vi "Execute.vi"(8 "error in (no error)":errorcluster, 10 "Notify Plugin Slide Completed in":refnum<class "Notify Plugin Slide Completed.lvclass">, 11 "Plugin Handler Shifter Data Definition":T1) -> (0 "error out":errorcluster, 1 "Stop?":bool, 2 "Plugin Generic Command out":refnum<class "Plugin Handler Command.lvclass">, 3 "Plugin Handler Shifter Data Out":T1)   [LabVIEW 2011, in "Notify Plugin Slide Completed.lvclass"]
uses:
  Notify Plugin Slide Completed.lvclass
  Plugin Handler Command.lvclass
  Plugin Strict Type Definitions/Plugin Handler Shifter Data Definition.ctl
  Parent Plugin Definition/Plugin Template/Generic Plugin.lvclass
  Plugin Strict Type Definitions/Plugin Configuration Information.ctl
  User Interface/UI Command Manager/UI Command Manager.lvclass
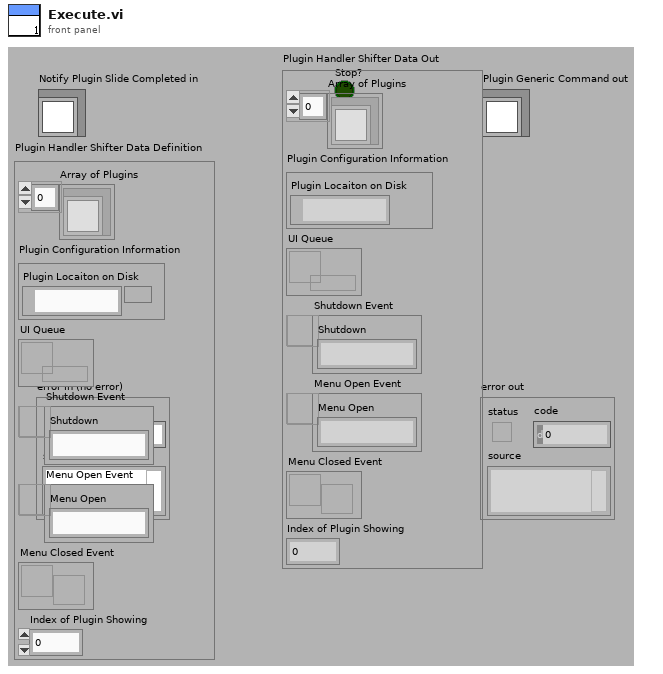
[diagram p1: front panel]
types:
  T1 = typedef "Plugin Handler Shifter Data Definition.ctl" = cluster{"Array of Plugins":refnum<class "Generic Plugin.lvclass">[], "Plugin Configuration Information":T2, "UI Queue":refnum<queue>, "Shutdown Event":refnum<user-event>, "Menu Open Event":refnum<user-event>, "Menu Closed Event":refnum<user-event>, "Index of Plugin Showing":i32}
  T2 = typedef "Plugin Configuration Information.ctl" = cluster{"Plugin Locaiton on Disk":path}
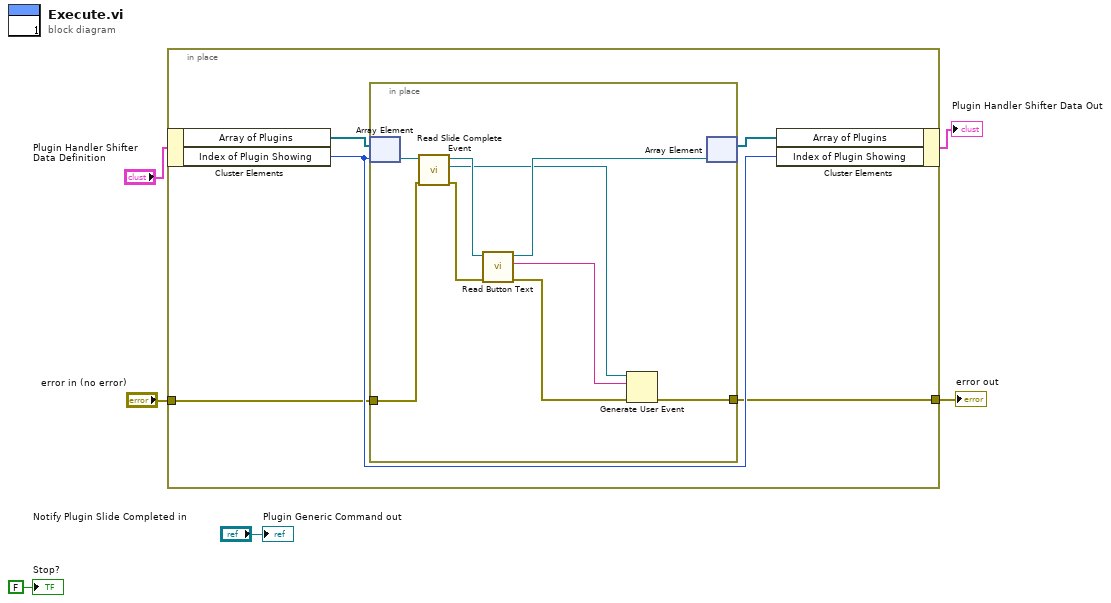
[diagram p0: block diagram]
diagram:
  n1 = in-place {
    in-place-border: "error in (no error)" -> [w8]
    in-place-border: [w7] -> w3
    n2 = in-place-cluster #1("Plugin Handler Shifter Data Definition") -> ("Array of Plugins"=w11:refnum<class "Generic Plugin.lvclass">[], "Index of Plugin Showing"=w9:i32)
    n3 = in-place {
      in-place-border: w8 -> [w17]
      in-place-border: [w12] -> w7
      n4 = in-place-array #2(w11, w9) -> (w20:refnum<class "Generic Plugin.lvclass">)
      n5 = call "Read Slide Complete Event.vi"("error in (no error)"=w17, "Generic Plugin in"=w20) -> ("error out"=w16:errorcluster, "Slide Complete Event"=w14:refnum<user-event>, "Generic Plugin out"=w19:refnum<class "Generic Plugin.lvclass">)  [unwired: 7 in]
      n6 = call-dynamic "Read Button Text.vi"("error in (no error)"=w16, "Generic Plugin in"=w19) -> ("error out"=w13:errorcluster, "Button Text"=w15:string, "Generic Plugin out"=w18:refnum<class "Generic Plugin.lvclass">)  [unwired: 7 in]
      n7 = Generate User Event(user event=w14, event data cluster=w15, error in=w13) -> (error out=w12:errorcluster)  [unwired: 1 out]
      n8 = in-place-array #2(w18) -> (w10:refnum<class "Generic Plugin.lvclass">[])  [unwired: 1 out]
    }
    n9 = in-place-cluster #1("Array of Plugins"=w10, "Index of Plugin Showing"=w9) -> (→"Plugin Handler Shifter Data Out":T1)
  }
  "error out" <- w3
  "Plugin Generic Command out" <- "Notify Plugin Slide Completed in"
  "Stop?" <- FALSE ("Stop?")
